vi "Write_occurrence.vi"(0 "Without data DVR reference in":refnum<data-value>, 5 "Occurrence Ref":refnum<k4>, 11 "error in (no error)":errorcluster) -> (4 "Without data DVR reference out":refnum<data-value>, 15 "error out":errorcluster)   [LabVIEW 2020, in "Data Communication Transmitter.lvlib" / "Without Data.lvclass"]
doc: "This VI is the parent which is used to write the occurrence reference to the DVR"
uses:
  Classes/Children/Intra-Application/Children/Without data/Without Data.lvclass
  Classes/Children/Intra-Application/Children/Without data/Without Data.lvclass/Without Data.ctl
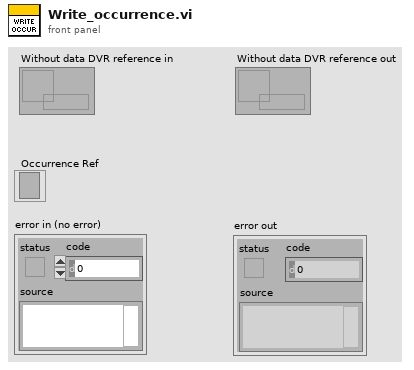
[diagram p1: front panel]
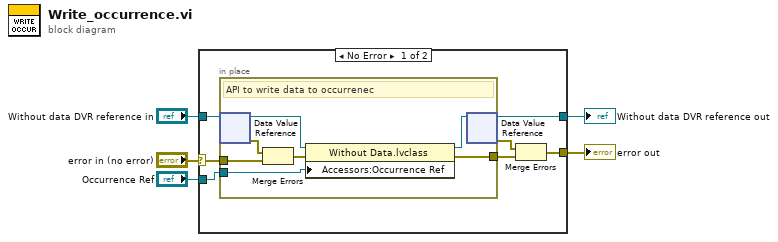
[diagram p0: block diagram]
diagram:
  n1 = case shown="No Error" "error in (no error)" {
    selector: "error in (no error)" -> [w10 w21]
    tunnel: [w6 w21] -> w4
    tunnel: "Without data DVR reference in" -> [w12 w20]
    tunnel: [w11 w20] -> w2
    tunnel: "Occurrence Ref" -> [w9 _]
    frame No Error {
      n2 = in-place "In Place Element Structure" {
        in-place-border: w10 -> [w16]
        in-place-border: w9 -> [w18]
        in-place-border: [w13] -> w8
        # "API to write data to occurrenec"
        n3 = in-place-dvr #1(w12) -> (w19:refnum<class "Without Data.lvclass">, w15:errorcluster)
        n4 = Merge Errors(w15, w16) -> (w17:errorcluster)
        n5 = property on="Property Node" class="Without Data.lvclass"(reference=w19, error in=w17, "Accessors:Occurrence Ref"=w18) -> (reference out=w14:refnum<class "Without Data.lvclass">, error out=w13:errorcluster)
        n6 = in-place-dvr #1(w14) -> (w11:refnum<data-value>, w7:errorcluster)
      }
      n7 = Merge Errors(w7, w8) -> (w6:errorcluster)
    }
    frame Error {
    }
  }
  "error out" <- w4
  "Without data DVR reference out" <- w2
